vi "led A.vi"() -> ()   [LabVIEW 2012]
uses:
  <vilib>/FieldPoint/Polymorphic Write.llb/FP Write (Float -IO).vi
panel:
  out "x-y*floor(x/y)":i32
  in  "FieldPoint IO Point":refnum<k21>="FieldPoint\\NI-cFP2220-0165C974\\cFP-2220 @0\\LED A"
  in  "stop":bool
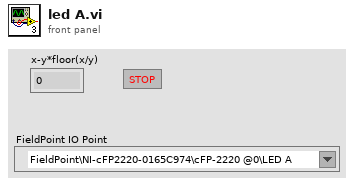
[diagram p1: front panel]
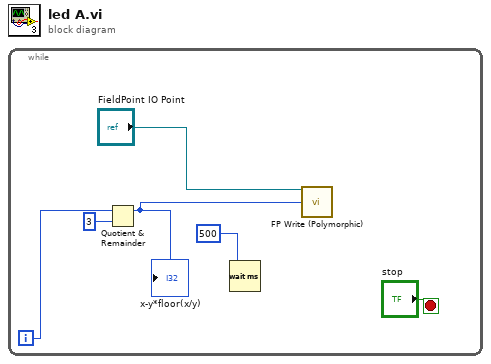
[diagram p0: block diagram]
diagram:
  n1 = while {
    i -> [w4]
    stop <- "stop" stop-if-true
    n2 = Quotient & Remainder(x=w4, y=3) -> (x-y*floor(x/y)=w2:i32)  [unwired: 1 out]
    "x-y*floor(x/y)" <- w2
    n3 = Wait (ms)(milliseconds to wait=u32 500) -> ()  [unwired: 1 out]
    n4 = call-poly <vilib>:"FP Write (Polymorphic).vi"("FieldPoint IO Point In"="FieldPoint IO Point", "value"=w2) -> ()  [unwired: 11 in, 3 out]
  }
